vi "Actor Core.vi"(8 "error in":errorcluster, 11 "Signal_Gen in":refnum<class "Signal_Gen.lvclass">) -> (0 "error out":errorcluster, 3 "Actor out":refnum<class "Actor.lvclass">)   [LabVIEW 2019, in "Signal_Gen.lvlib" / "Signal_Gen.lvclass"]
doc: "(<B>Filename</B>: Actor Framework.lvlib:Actor.lvclass:Actor Core.vi)\n\nReceives messages to the actor, reacts to them, and initiates any error handling that may shut the actor down.\n\nDescendant classes may override this VI to append parallel tasks for the actor to complete while it handles messages. Overrides use the Call Parent Method node."
uses:
  Signal_Gen.lvclass
  C:/Program Files/National Instruments/LabVIEW 2019/vi.lib/ActorFramework/Actor/Actor.lvclass
  <vilib>/ActorFramework/Actor/Actor.lvclass
  <vilib>/ActorFramework/Actor/Actor.lvclass/Actor.ctl
  Signal_Gen.lvclass/Signal_Gen.ctl
  GUI_Actor Messages/Graph_signal Msg/Graph_signal Msg.lvclass/Graph_signal Msg.ctl
  <vilib>/ActorFramework/Message Enqueuer/Message Enqueuer.lvclass/Message Enqueuer.ctl
  <vilib>/ActorFramework/Message Enqueuer/Enqueue.vi
  GUI_Actor Messages/Graph_signal Msg/Graph_signal Msg.lvclass
  C:/Program Files/National Instruments/LabVIEW 2019/vi.lib/ActorFramework/Message/Message.lvclass
  <vilib>/ActorFramework/Stop Msg/Stop Msg.lvclass
  <vilib>/ActorFramework/Message Priority Queue/Priority Enqueue.vi
  <vilib>/measure/NI_MABase.lvlib
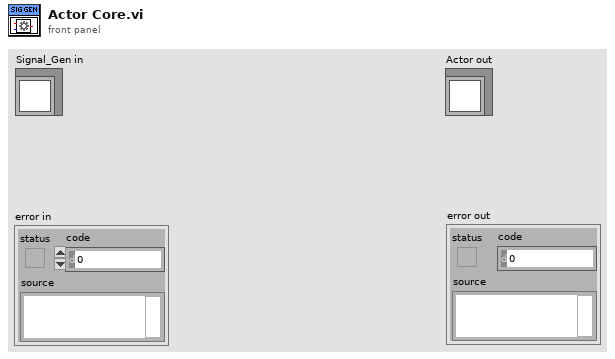
[diagram p1: front panel]
types:
  T1 = cluster{"Start/Stop":refnum<user-event>, "Exit":refnum<user-event>, "Tipo de señal":refnum<user-event>, "Amplitud":refnum<user-event>, "Frecuencia":refnum<user-event>}
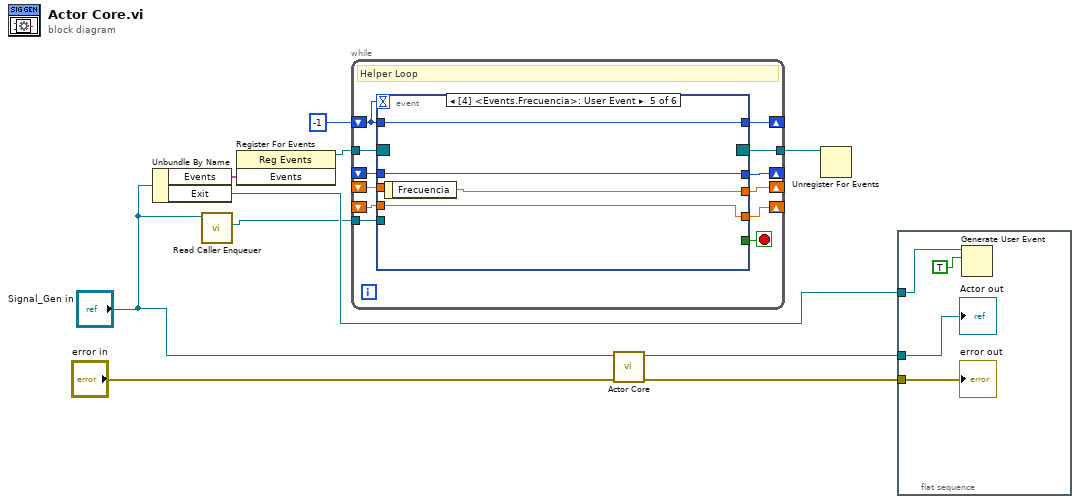
[diagram p0: block diagram]
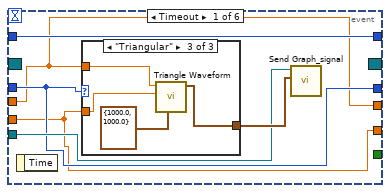
[diagram p2: hidden frame]
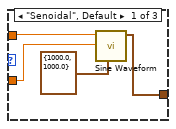
[diagram p3: hidden frame]
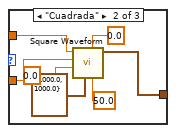
[diagram p4: hidden frame]
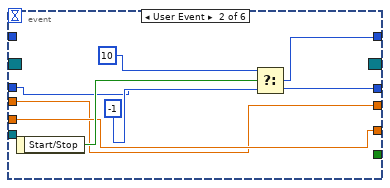
[diagram p5: hidden frame]
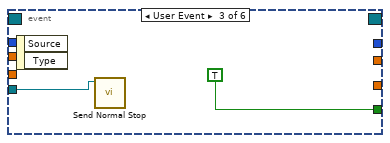
[diagram p6: hidden frame]
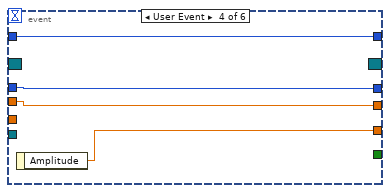
[diagram p7: hidden frame]
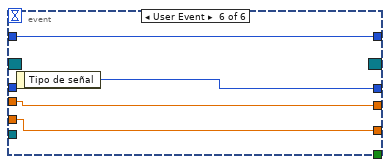
[diagram p8: hidden frame]
diagram:
  n1 = Unbundle By Name("Signal_Gen in") -> ("Events"=w6:T1, "Exit"=w3:refnum<user-event>)
  n2 = call <vilib>:"Read Caller Enqueuer.vi"("Actor"="Signal_Gen in") -> ("Caller Enqueuer"=w1:refnum<class "Message Enqueuer.lvclass">)  [unwired: 10 in]
  n3 = register-events(w6) -> (reference out=w5:refnum<event-registration>)  [unwired: 2 in, 1 out]
  n4 = while {
    shift-right: [w22] -> _
    shift-left: -1 -> [w17]
    tunnel: w5 -> [w21]
    tunnel: [w20] -> w4
    tunnel: w1 -> [w18]
    shift-right: [w16] -> _
    shift-left: _ -> [w15]
    shift-right: [w14] -> _
    shift-left: _ -> [w13]
    shift-right: [w12] -> _
    shift-left: _ -> [w11]
    stop <- w19 stop-if-true
    # "Helper Loop"
    n5 = event shown="[4] <Events.Frecuencia>: User Event" {
      selector: w21 -> [_ _ _ _ _ _]
      dyn-events: [_ _ _ _ _ _] -> w20
      timeout: w17 -> [_ _ _ _ _ _]
      tunnel: w17 -> [w28 _ _ w53 w57 w62]
      tunnel: [w28 w47 _ w53 w57 w62] -> w22
      tunnel: [_ _ TRUE _ _ _] -> w19
      tunnel: w18 -> [w26 _ w51 _ _ _]
      tunnel: [w25 w46 _ w55 w59 w64] -> w16
      tunnel: w15 -> [w25 w46 _ w55 w59 _]
      tunnel: [w24 w45 _ w56 w58 w63] -> w14
      tunnel: w13 -> [w24 w45 _ _ w58 w63]
      tunnel: [w23 w44 _ w54 w60 w61] -> w12
      tunnel: w11 -> [w23 w44 _ w54 _ w61]
      event Timeout {
        n6 = event-data() -> ()  [unwired: 1 in, 1 out]
        n7 = case shown="\"Triangular\"" w25 {
          tunnel: [w31 w35 w42] -> w27
          tunnel: w24 -> [w30 w34 w41]
          tunnel: w23 -> [w29 w33 w40]
          frame "Senoidal", Default {
            n8 = call <vilib>:"Sine Waveform.vi"("sampling info"=cluster{"Fs":dbl, "#s":dbl} {"Fs"=1000.0, "#s"=1000.0}, "amplitude"=w30, "frequency"=w29) -> ("signal out"=w31:waveform(dbl))  [unwired: 7 in, 1 out]
          }
          frame "Cuadrada" {
            n9 = call <vilib>:"Square Waveform.vi"("duty cycle (%)"=50.0, "offset"=0.0, "sampling info"=cluster{"Fs":dbl, "#s":dbl} {"Fs"=1000.0, "#s"=1000.0}, "phase"=0.0, "amplitude"=w34, "frequency"=w33) -> ("signal out"=w35:waveform(dbl))  [unwired: 4 in, 1 out]
          }
          frame "Triangular" {
            n10 = call <vilib>:"Triangle Waveform.vi"("sampling info"=cluster{"Fs":dbl, "#s":dbl} {"Fs"=1000.0, "#s"=1000.0}, "amplitude"=w41, "frequency"=w40) -> ("signal out"=w42:waveform(dbl))  [unwired: 7 in, 1 out]
          }
        }
        n11 = call "Send Graph_signal.vi"("Grafica"=w27, "Message Enqueuer"=w26) -> ()  [unwired: 8 in, 2 out]
      }
      event User Event {
        n12 = event-data() -> ("Start/Stop"=w50:bool)  [unwired: 1 in]
        n13 = Select(t=10, s=w50, f=-1) -> (s? t:f=w47:i32)
      }
      event User Event {
        n14 = event-data() -> ()  [unwired: 1 in, 2 out]
        n15 = call <vilib>:"Send Normal Stop.vi"("Message Enqueuer"=w51) -> ()  [unwired: 10 in, 1 out]
      }
      event User Event {
        n16 = event-data() -> ("Amplitude"=w56:dbl)  [unwired: 1 in]
      }
      event User Event {
        n17 = event-data() -> ("Frecuencia"=w60:dbl)  [unwired: 1 in]
      }
      event User Event {
        n18 = event-data() -> ("Tipo de señal"=w64:enum16{"Senoidal", "Cuadrada", "Triangular"})  [unwired: 1 in]
      }
    }
  }
  n19 = call-parent "Actor Core.vi"("error in"="error in", "Actor in"="Signal_Gen in") -> ("error out"=w10:errorcluster, "Actor out"=w9:refnum<class "Actor.lvclass">)  [unwired: 8 in]
  n20 = Unregister For Events(event registration refnum=w4) -> ()  [unwired: 1 in, 1 out]
  n21 = flat-sequence {
    tunnel: w10 -> [w68]
    tunnel: w9 -> [w67]
    tunnel: w3 -> [w66]
    frame #0 {
      n22 = Generate User Event(user event=w66, event data cluster=TRUE ("event data")) -> ()  [unwired: 2 in, 2 out]
      "error out" <- w68
      "Actor out" <- w67
    }
  }
